vi "Needle Voltage.vi"(10 "Action":T1, 11 "Input Needle Voltage":dbl) -> (3 "Output Needle Voltage":dbl)   [LabVIEW 2013]
uses:
  Functional Global Variables/Action Items.ctl
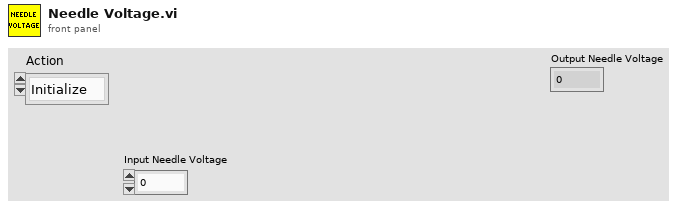
[diagram p1: front panel]
types:
  T1 = typedef "Action Items.ctl" = enum16{"Initialize", "Get", "Set"}
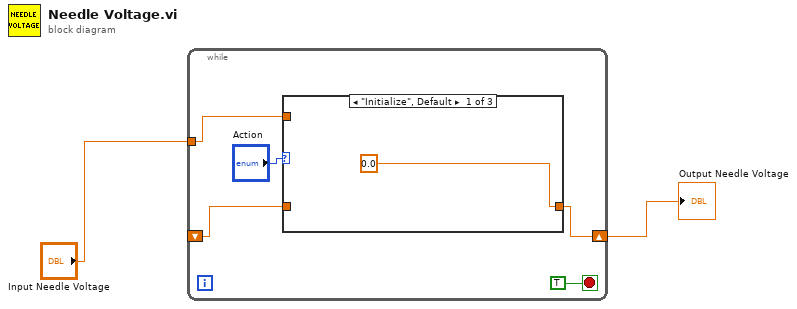
[diagram p0: block diagram]
diagram:
  n1 = while {
    shift-right: [w4] -> w1
    shift-left: _ -> [w5]
    tunnel: "Input Needle Voltage" -> [w6]
    stop <- TRUE stop-if-true
    n2 = case shown="\"Initialize\", Default" "Action" {
      tunnel: w6 -> [_ w9 _]
      tunnel: [0.0 w9 w10] -> w4
      tunnel: w5 -> [_ _ w10]
      frame "Initialize", Default {
      }
      frame "Set" {
      }
      frame "Get" {
      }
    }
  }
  "Output Needle Voltage" <- w1
